vi "VI Checksum.vi"(10 "VI":refnum<vi>) -> (2 "VI Checksum":string)   [LabVIEW 2015, in "Message Maker.lvclass"]
doc: "Generates a checksum for the VI based on it's block diagram contents, description and icon\n\nAuthor: Derek Trepanier\nCopyright: MGI 2015"
uses:
  Message Maker.lvclass
  <vilib>/Utility/traverseref.llb/TRef TravTarget.ctl
  <vilib>/Utility/traverseref.llb/VI Scripting - Traverse.lvlib
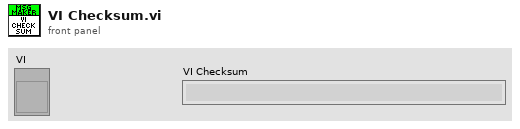
[diagram p1: front panel]
types:
  T1 = typedef "TRef TravTarget.ctl" = enum16{"FP", "BD", "Other"}
  T2 = typedef "imagedata.ctl" = cluster{"image type":i32, "image depth":i32, "image":u8[], "mask":u8[], "colors":u32[], "Rectangle":cluster{"left":i16, "top":i16, "right":i16, "bottom":i16}}
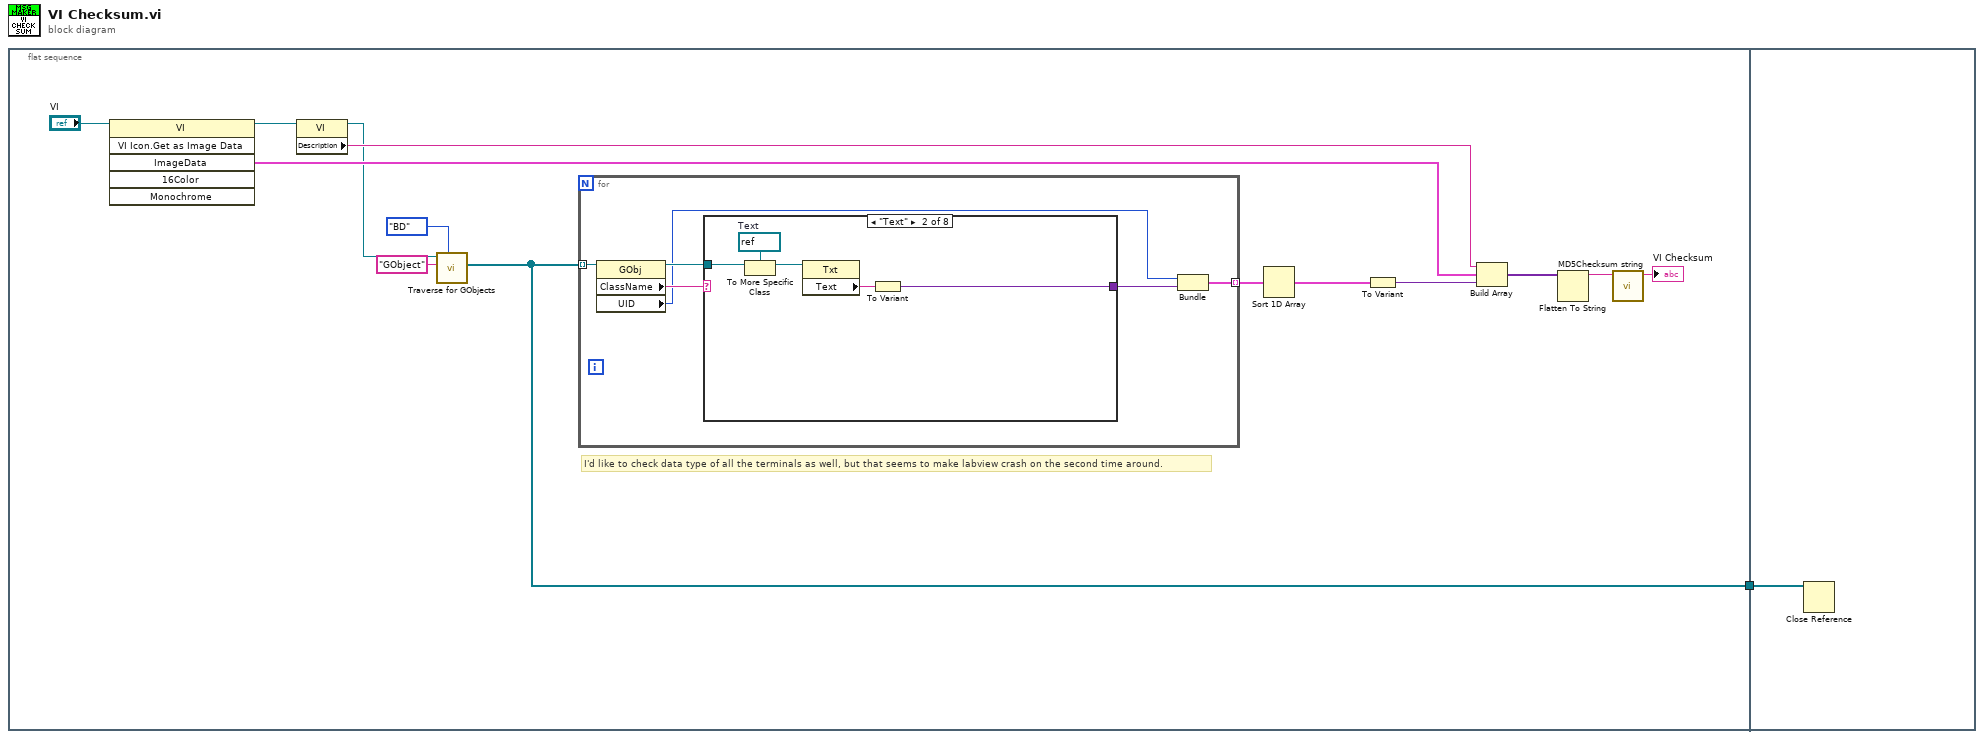
[diagram p0: block diagram]
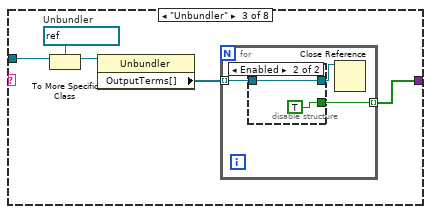
[diagram p3: hidden frame]
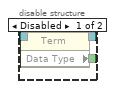
[diagram p4: hidden frame]
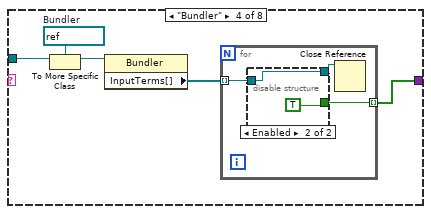
[diagram p5: hidden frame]
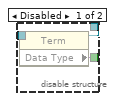
[diagram p6: hidden frame]
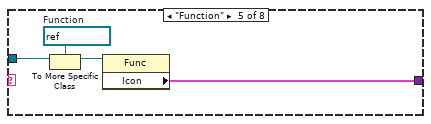
[diagram p7: hidden frame]
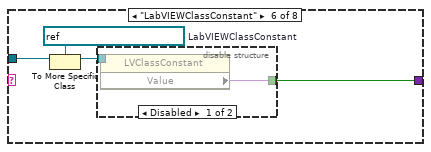
[diagram p8: hidden frame]
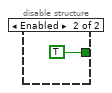
[diagram p9: hidden frame]
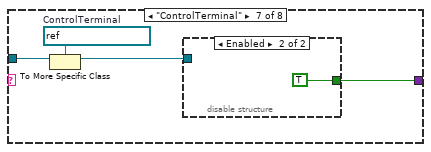
[diagram p10: hidden frame]
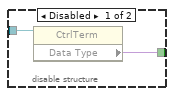
[diagram p11: hidden frame]
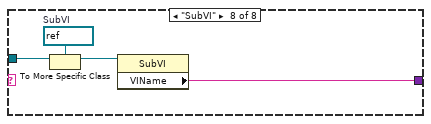
[diagram p12: hidden frame]
diagram:
  n1 = flat-sequence {
    tunnel: [w8] -> w1
    tunnel: w1 -> [w75]
    frame #0 {
      # "I'd like to check data type of all the terminals as well, but that seems to make labview crash on the second time around."
      n2 = invoke class="VI" method="VI Icon.Get as Image Data"(reference="VI") -> (reference out=w13:refnum<vi>, "ImageData"=w11:T2)  [unwired: 5 in, 4 out]
      n3 = property class="VI"(reference=w13) -> (reference out=w9:refnum<vi>, "Description"=w12:string)  [unwired: 1 in, 1 out]
      n4 = call <vilib>:"Traverse for GObjects.vi"("Traverse Target"=TRef_TravTarget."BD", "Class Name"="GObject", "VI Refnum"=w9) -> ("References"=w8:refnum<vi>[])  [unwired: 5 in, 3 out]
      n5 = for {
        tunnel: w8 -> [w21] mode=indexing
        tunnel: [w16] -> w10 mode=indexing
        n6 = property class="GObj"(reference=w21) -> (reference out=w19:refnum<vi>, "ClassName"=w20:string, "UID"=w17:i32)  [unwired: 1 in, 1 out]
        n7 = case shown="\"Text\"" w20 {
          tunnel: w19 -> [_ w25 w30 w43 w55 w59 w66 w73]
          tunnel: [_ w22 w27 w40 w53 w58 w64 w71] -> w18
          frame Default {
          }
          frame "Text" {
            w26 = refnum<vi> refnum  # Text
            n8 = To More Specific Class(target class=w26, reference=w25) -> (specific class reference=w24:refnum<vi>)  [unwired: 1 in, 1 out]
            n9 = property class="Txt"(reference=w24) -> ("Text"=w23:string)  [unwired: 1 in, 2 out]
            n10 = To Variant(anything=w23) -> (Variant=w22:variant)
          }
          frame "Unbundler" {
            w31 = refnum<vi> refnum  # Unbundler
            n11 = To More Specific Class(target class=w31, reference=w30) -> (specific class reference=w29:refnum<vi>)  [unwired: 1 in, 1 out]
            n12 = property class="Unbundler"(reference=w29) -> ("OutputTerms[]"=w28:refnum<vi>[])  [unwired: 1 in, 2 out]
            n13 = for {
              tunnel: w28 -> [w34] mode=indexing
              tunnel: [w33] -> w27 mode=indexing
              n14 = disable-structure shown="Enabled" {
                disable-tunnel: w34 -> [w37 w39]
                disable-tunnel: [w36 TRUE] -> w33
                disable-tunnel: [w35 w39] -> w32
                frame Disabled {
                  n15 = property class="Term"(reference=w37) -> (reference out=w35:refnum<vi>, "Data Type"=w36:variant)  [unwired: 1 in, 1 out]
                }
                frame Enabled {
                }
              }
              n16 = Close Reference(reference=w32) -> ()  [unwired: 1 in, 1 out]
            }
          }
          frame "Bundler" {
            w44 = refnum<vi> refnum  # Bundler
            n17 = To More Specific Class(target class=w44, reference=w43) -> (specific class reference=w42:refnum<vi>)  [unwired: 1 in, 1 out]
            n18 = property class="Bundler"(reference=w42) -> ("InputTerms[]"=w41:refnum<vi>[])  [unwired: 1 in, 2 out]
            n19 = for {
              tunnel: w41 -> [w47] mode=indexing
              tunnel: [w46] -> w40 mode=indexing
              n20 = disable-structure shown="Enabled" {
                disable-tunnel: w47 -> [w50 w52]
                disable-tunnel: [w49 TRUE] -> w46
                disable-tunnel: [w48 w52] -> w45
                frame Disabled {
                  n21 = property class="Term"(reference=w50) -> (reference out=w48:refnum<vi>, "Data Type"=w49:variant)  [unwired: 1 in, 1 out]
                }
                frame Enabled {
                }
              }
              n22 = Close Reference(reference=w45) -> ()  [unwired: 1 in, 1 out]
            }
          }
          frame "Function" {
            w56 = refnum<vi> refnum  # Function
            n23 = To More Specific Class(target class=w56, reference=w55) -> (specific class reference=w54:refnum<vi>)  [unwired: 1 in, 1 out]
            n24 = property class="Func"(reference=w54) -> ("Icon"=w53:T2)  [unwired: 1 in, 2 out]
          }
          frame "LabVIEWClassConstant" {
            w60 = refnum<vi> refnum  # LabVIEWClassConstant
            n25 = To More Specific Class(target class=w60, reference=w59) -> (specific class reference=w57:refnum<vi>)  [unwired: 1 in, 1 out]
            n26 = disable-structure shown="Disabled" {
              disable-tunnel: [w62 TRUE] -> w58
              disable-tunnel: w57 -> [w61 _]
              frame Disabled {
                n27 = property class="LVClassConstant"(reference=w61) -> ("Value"=w62:variant)  [unwired: 1 in, 2 out]
              }
              frame Enabled {
              }
            }
          }
          frame "ControlTerminal" {
            w67 = refnum<vi> refnum  # ControlTerminal
            n28 = To More Specific Class(target class=w67, reference=w66) -> (specific class reference=w65:refnum<vi>)  [unwired: 1 in, 1 out]
            n29 = disable-structure shown="Enabled" {
              disable-tunnel: w65 -> [w69 _]
              disable-tunnel: [w68 TRUE] -> w64
              frame Disabled {
                n30 = property class="CtrlTerm"(reference=w69) -> ("Data Type"=w68:variant)  [unwired: 1 in, 2 out]
              }
              frame Enabled {
              }
            }
          }
          frame "SubVI" {
            w74 = refnum<vi> refnum  # SubVI
            n31 = To More Specific Class(target class=w74, reference=w73) -> (specific class reference=w72:refnum<vi>)  [unwired: 1 in, 1 out]
            n32 = property class="SubVI"(reference=w72) -> ("VIName"=w71:string)  [unwired: 1 in, 2 out]
          }
        }
        n33 = Bundle("UID"=w17, "Variant"=w18) -> (w16:cluster{"UID":i32, "Variant":variant})  [unwired: 1 in]
      }
      n34 = Sort 1D Array(array=w10) -> (sorted array=w5:cluster{"UID":i32, "Variant":variant}[])
      n35 = To Variant(anything=w5) -> (Variant=w4:variant)
      n36 = Build Array(w12, w11, w4) -> (w2:variant[])
      n37 = Flatten To String(anything=w2) -> (data string=w15:string)  [unwired: 3 in, 2 out]
      n38 = call <vilib>:"MD5Checksum string.vi"("Message String"=w15) -> ("MD5 message-digest"=→"VI Checksum":string)  [unwired: 10 in]
    }
    frame #1 {
      n39 = Close Reference(reference=w75) -> ()  [unwired: 1 in, 1 out]
    }
  }
